vi "Launch Element.vi"() -> ()   [LabVIEW 2016]
uses:
  Sequence Element.lvclass
  D:/Program Files/National Instruments/LabVIEW 2016/vi.lib/ActorFramework/Actor/Actor.lvclass
  <vilib>/ActorFramework/Message Enqueuer/Message Enqueuer.lvclass/Message Enqueuer.ctl
  Sequence Element Messages/Add Items Msg/Add Items Msg.lvclass/Add Items Msg.ctl
  <vilib>/ActorFramework/Message Enqueuer/Enqueue.vi
  Da Base Messages/Open Front Panel Msg/Open Front Panel Msg.lvclass
  D:/Program Files/National Instruments/LabVIEW 2016/vi.lib/ActorFramework/Message/Message.lvclass
  Sequence Element Messages/Add Items Msg/Add Items Msg.lvclass
  <vilib>/ActorFramework/Stop Msg/Stop Msg.lvclass
  <vilib>/ActorFramework/Message Priority Queue/Priority Enqueue.vi
  <vilib>/ActorFramework/Actor/Actor.lvclass
panel:
  in  "Items":string[](array[string])=["RP sweep", "Cryo-con"]
  in  "Stop Button":bool
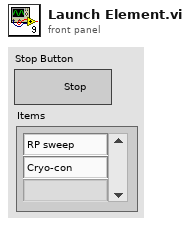
[diagram p1: front panel]
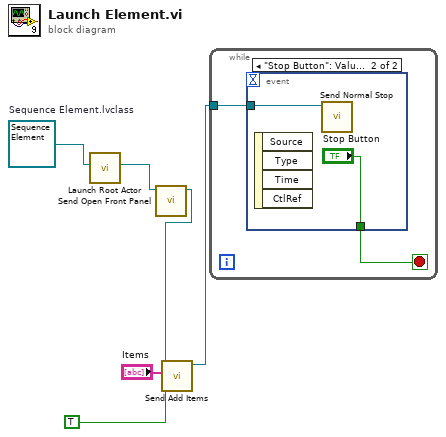
[diagram p0: block diagram]
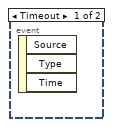
[diagram p2: hidden frame]
diagram:
  w6 = refnum<class "Sequence Element.lvclass"> refnum  # Sequence Element.lvclass
  n1 = call <vilib>:"Launch Root Actor.vi"("Actor"=w6) -> ("Actor's Enqueuer"=w5:refnum<class "Message Enqueuer.lvclass">)  [unwired: 9 in, 1 out]
  n2 = call "Send Open Front Panel.vi"("Message Enqueuer"=w5) -> ("Message Enqueuer out"=w3:refnum<class "Message Enqueuer.lvclass">)  [unwired: 9 in, 1 out]
  n3 = call "Send Add Items.vi"("Reset"=TRUE, "Items"="Items", "Message Enqueuer"=w3) -> ("Message Enqueuer out"=w2:refnum<class "Message Enqueuer.lvclass">)  [unwired: 7 in, 1 out]
  n4 = while {
    tunnel: w2 -> [w7]
    stop <- w8 stop-if-true
    n5 = event shown="[1] \"Stop Button\": Value Change" {
      selector: _ -> [_ _]
      dyn-events: _ -> [_ _]
      timeout: _ -> [_ _]
      tunnel: [_ "Stop Button"] -> w8
      tunnel: w7 -> [_ w9]
      event Timeout {
        n6 = event-data() -> ()  [unwired: 1 in, 3 out]
      }
      event "Stop Button": Value Change {
        n7 = event-data() -> ()  [unwired: 1 in, 4 out]
        n8 = call <vilib>:"Send Normal Stop.vi"("Message Enqueuer"=w9) -> ()  [unwired: 10 in, 1 out]
      }
    }
  }
